vi "set_relay.vi"(6 "ch_4":bool, 8 "ch_3":bool, 9 "ch_2":bool, 10 "ch_1":bool, 11 "Handle":u64) -> (0 "message":string, 1 "ch_2_out":bool, 2 "ch_1_out":bool, 3 "Handle_out":u64, 4 "status":bool)   [LabVIEW 2019]
panel:
  out "bytes_wait":u32
  out "bytes_written":u32
  out "status_read":u32(ring) items=["FT_OK", "FT_INVALID_HANDLE", "FT_DEVICE_NOT_FOUND", "FT_DEVICE_NOT_OPENED", "FT_IO_ERROR", "FT_INSUFFICIENT_RESOURCES", "FT_INVALID_PARAMETER", "FT_INVALID_BAUD_RATE", "FT_DEVICE_NOT_OPENED_FOR_ERASE", "FT_DEVICE_NOT_OPENED_FOR_WRITE", "FT_FAILED_TO_WRITE_DEVICE", "FT_EEPROM_READ_FAILED", "FT_EEPROM_WRITE_FAILED", "FT_EEPROM_ERASE_FAILED", "FT_EEPROM_NOT_PRESENT", "FT_EEPROM_NOT_PROGRAMMED", "FT_INVALID_ARGS", "FT_NOT_SUPPORTED", "FT_OTHER_ERROR"]
  out "status_write":u32(ring) items=["FT_OK", "FT_INVALID_HANDLE", "FT_DEVICE_NOT_FOUND", "FT_DEVICE_NOT_OPENED", "FT_IO_ERROR", "FT_INSUFFICIENT_RESOURCES", "FT_INVALID_PARAMETER", "FT_INVALID_BAUD_RATE", "FT_DEVICE_NOT_OPENED_FOR_ERASE", "FT_DEVICE_NOT_OPENED_FOR_WRITE", "FT_FAILED_TO_WRITE_DEVICE", "FT_EEPROM_READ_FAILED", "FT_EEPROM_WRITE_FAILED", "FT_EEPROM_ERASE_FAILED", "FT_EEPROM_NOT_PRESENT", "FT_EEPROM_NOT_PROGRAMMED", "FT_INVALID_ARGS", "FT_NOT_SUPPORTED", "FT_OTHER_ERROR"]
  out "string_write":string
  out "channel_bits":u8=1 max=15
  out "string_read":string
  out "bytes_read":u32
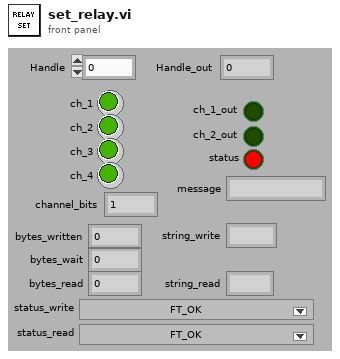
[diagram p1: front panel]
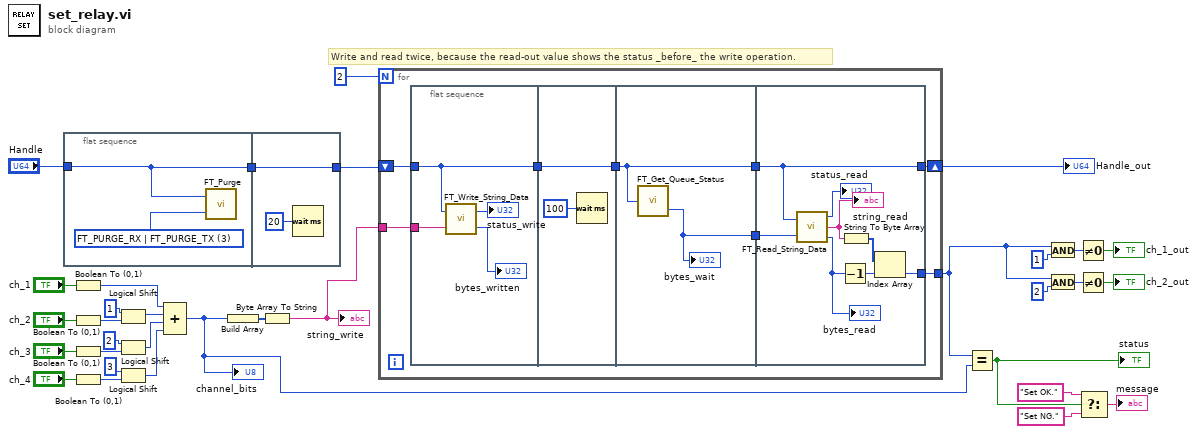
[diagram p0: block diagram]
diagram:
  # "Write and read twice, because the read-out value shows the status _before_ the write operation."
  n1 = flat-sequence {
    tunnel: "Handle" -> [w34]
    tunnel: [w34] -> w8
    tunnel: w8 -> [w36]
    tunnel: [w36] -> w7
    frame #0 {
      w35 = u32 3 items=["FT_PURGE_RX"=1, "FT_PURGE_TX"=2, "FT_PURGE_RX | FT_PURGE_TX"=3] ("Purge Flags")
      n2 = call "FT_Purge.vi"("Purge Flags"=w35, "Handle"=w34) -> ()  [unwired: 1 out]
    }
    frame #1 {
      n3 = Wait (ms)(milliseconds to wait=u32 20) -> ()  [unwired: 1 out]
    }
  }
  n4 = Boolean To (0,1)(Boolean="ch_1") -> (0, 1=w23:i16)
  n5 = Boolean To (0,1)(Boolean="ch_2") -> (0, 1=w29:i16)
  n6 = Boolean To (0,1)(Boolean="ch_3") -> (0, 1=w27:i16)
  n7 = Boolean To (0,1)(Boolean="ch_4") -> (0, 1=w26:i16)
  n8 = Logical Shift(y=i16 1, x=w29) -> (x << y=w22:i16)
  n9 = Logical Shift(y=i16 2, x=w27) -> (x << y=w21:i16)
  n10 = Logical Shift(y=i16 3, x=w26) -> (x << y=w20:i16)
  n11 = Compound Arithmetic op=ADD(w23, w22, w21, w20) -> (w5:i16)
  "channel_bits" <- w5
  n12 = Build Array(w5) -> (w19:i16[])
  n13 = Byte Array To String(unsigned byte array=w19) -> (string=w16:string)
  "string_write" <- w16
  n14 = for {
    N: 2 -> [_]
    tunnel: w16 -> [w43]
    shift-right: [w42] -> w17
    shift-left: w7 -> [w44]
    tunnel: [w38] -> w6
    n15 = flat-sequence {
      tunnel: w44 -> [w47]
      tunnel: w43 -> [w48]
      tunnel: [w47] -> w45
      tunnel: [w50] -> w41
      tunnel: w45 -> [w50]
      tunnel: w41 -> [w53]
      tunnel: [w53] -> w40
      tunnel: [w52] -> w39
      tunnel: w40 -> [w60]
      tunnel: [w60] -> w42
      tunnel: w39 -> [w59]
      tunnel: [w54] -> w38
      frame #0 {
        n16 = call "FT_Write_String_Data.vi"("Buffer"=w48, "Handle"=w47) -> ("Bytes Written"=→"bytes_written":u32, "FT_Status"=→"status_write":u32)
      }
      frame #1 {
        n17 = Wait (ms)(milliseconds to wait=u32 100) -> ()  [unwired: 1 out]
      }
      frame #2 {
        n18 = call "FT_Get_Queue_Status.vi"("Handle"=w53) -> ("Bytes Waiting"=w52:u32)  [unwired: 1 out]
        "bytes_wait" <- w52
      }
      frame #3 {
        n19 = call "FT_Read_String_Data.vi"("Handle"=w60, "Bytes To Read"=w59) -> ("FT_Status"=→"status_read":u32, "Read Data"=w58:string, "Bytes Read"=w55:u32)
        "bytes_read" <- w55
        "string_read" <- w58
        n20 = Decrement(x=w55) -> (x-1=w56:u32)
        n21 = String To Byte Array(string=w58) -> (unsigned byte array=w57:u8[])
        n22 = Index Array(array=w57, index=w56) -> (element=w54:u8)
      }
    }
  }
  "Handle_out" <- w17
  n23 = Equal?(x=w6, y=w5) -> (x = y?=w4:bool)
  "status" <- w4
  n24 = And(x=w6, y=u32 1) -> (x .and. y?=w14:u32)
  n25 = And(x=w6, y=u32 2) -> (x .and. y?=w11:u32)
  n26 = Not Equal To 0?(x=w14) -> (x != 0?=→"ch_1_out":bool)
  n27 = Not Equal To 0?(x=w11) -> (x != 0?=→"ch_2_out":bool)
  n28 = Select(t="Set OK." ("message"), s=w4, f="Set NG." ("message")) -> (s? t:f=→"message":string)
